vi "ColorMap_GrayScale_LH.vi"(1 "Limits (L:0,H:255)":cluster{u8, u8}(slide)={0, 255} scale=0.0..255.0) -> (0 "GreyScale_LH":cluster{"Red":u8, "Green":u8, "Blue":u8}[](array[cluster]))   [LabVIEW 2012, in "HGF_VisionTools.lvlib"]
doc: "This VI calculates a rainbow color palette with low and high limits.\n\nDue to modulo operation the green colow in the middle may has 1-3 extra entries."
uses:
  HGF_VisionTools.lvlib
panel:
  in  "Color":cluster{"Red":u8, "Green":u8, "Blue":u8}
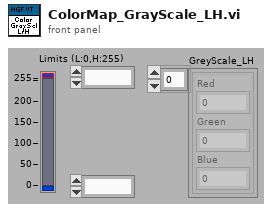
[diagram p1: front panel]
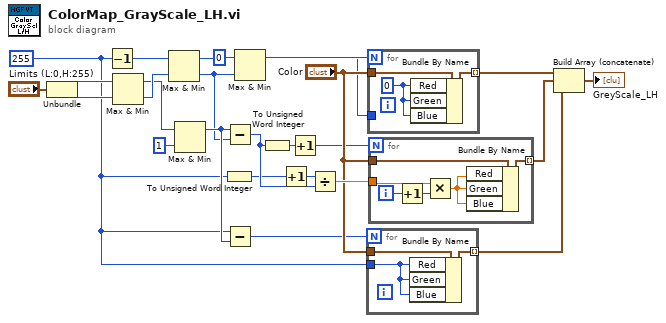
[diagram p0: block diagram]
diagram:
  w2 = u8 255 ("x")
  n1 = Unbundle("Limits (L:0,H:255)") -> (w17:u8, w16:u8)
  n2 = Decrement(x=w2) -> (x-1=w1:u8)
  n3 = Max & Min(x=w17, y=w16) -> (max(x,y)=w14:u8, min(x,y)=w15:u8)
  n4 = Max & Min(x=w1, y=w15) -> (min(x,y)=w13:u8)  [unwired: 1 out]
  n5 = Max & Min(x=w14, y=u8 1) -> (max(x,y)=w18:u8)  [unwired: 1 out]
  n6 = To Unsigned Word Integer(number=w2) -> (unsigned 16bit integer=w4:u16)
  n7 = Subtract(x=w18, y=w13) -> (x-y=w8:u8)
  n8 = Subtract(x=w2, y=w18) -> (x-y=w9:u8)
  n9 = Max & Min(x=u8 0, y=w13) -> (max(x,y)=w11:u8)  [unwired: 1 out]
  n10 = To Unsigned Word Integer(number=w8) -> (unsigned 16bit integer=w5:u16)
  n11 = Increment(x=w4) -> (x+1=w3:u16)
  n12 = Increment(x=w5) -> (x+1=w6:u16)
  n13 = Divide(x=w3, y=w8) -> (x/y=w20:dbl)
  n14 = for {
    N: w9 -> [_]
    tunnel: "Color" -> [w27]
    tunnel: [w26] -> w21 mode=indexing
    tunnel: w2 -> [w25]
    n15 = Bundle By Name(cluster=w27, "Red"=w25, "Green"=w25, "Blue"=w25) -> (w26:cluster{"Red":u8, "Green":u8, "Blue":u8})
  }
  n16 = for {
    N: w11 -> [_]
    tunnel: "Color" -> [w30]
    tunnel: [w29] -> w23 mode=indexing
    tunnel: w2 -> [_]
    w28 = u8 0 ("Green")
    n17 = Bundle By Name(cluster=w30, "Red"=w28, "Green"=w28, "Blue"=w28) -> (w29:cluster{"Red":u8, "Green":u8, "Blue":u8})
  }
  n18 = for {
    N: w6 -> [_]
    tunnel: "Color" -> [w36]
    tunnel: [w35] -> w22 mode=indexing
    tunnel: w20 -> [w34]
    i -> [w33]
    n19 = Increment(x=w33) -> (x+1=w32:i32)
    n20 = Multiply(x=w34, y=w32) -> (x*y=w31:dbl)
    n21 = Bundle By Name(cluster=w36, "Red"=w31, "Green"=w31, "Blue"=w31) -> (w35:cluster{"Red":u8, "Green":u8, "Blue":u8})
  }
  n22 = Build Array (concatenate)(w23, w22, w21) -> (→"GreyScale_LH":cluster{"Red":u8, "Green":u8, "Blue":u8}[])
